vi "average_LockIn.vi"(3 "error in":errorcluster, 4 "Count(mSec)":u32 caption="Sleep between measurements (mSec)", 5 "#AVG":dbl, 6 "Handle In":T2 {"Conn" format="0x%08x"}) -> (0 "Error Out":errorcluster, 1 "output cluster":T1, 2 "Handle Out":T2 {"Conn" format="0x%08x"})   [LabVIEW 2014]
uses:
  <instrlib>/Zurich Instruments LabOne/Public/ziTypeHandle.ctl
  <vilib>/express/express arith-compare/Formula/XNode/ExpressFormulaBlockNode.xnode
  <vilib>/Analysis/NI_AALBase.lvlib
  <instrlib>/Zurich Instruments LabOne/Zurich Instruments LabOne.lvlib
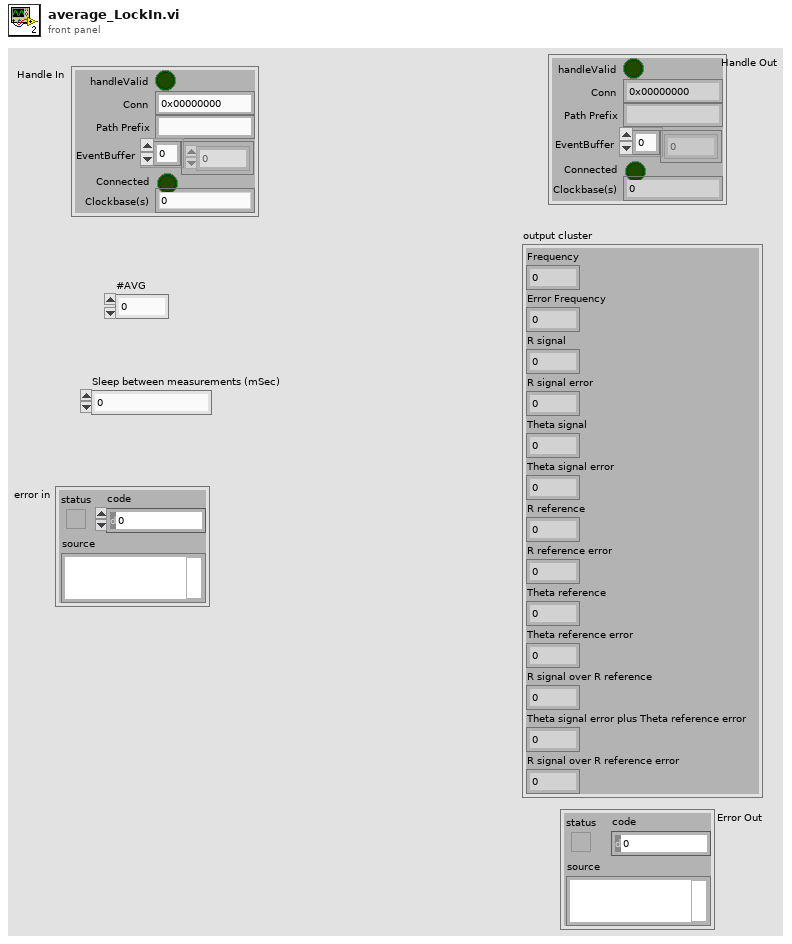
[diagram p1: front panel]
types:
  T1 = cluster{"Frequency":dbl, "Error Frequency ":dbl, "R signal":dbl, "R signal error":dbl, "Theta signal":dbl, "Theta signal error":dbl, "R reference":dbl, "R reference error":dbl, "Theta reference":dbl, "Theta reference error":dbl, "R signal over R reference":dbl, "Theta signal error plus Theta reference error":dbl, "R signal over R reference error":dbl}
  T2 = typedef "Zurich Instruments LabOne.lvlib/ziTypeHandle.ctl" = cluster{"handleValid":bool, "Conn":u64, "Path Prefix":string, "EventBuffer":u8[], "Connected":bool, "Clockbase(s)":dbl}
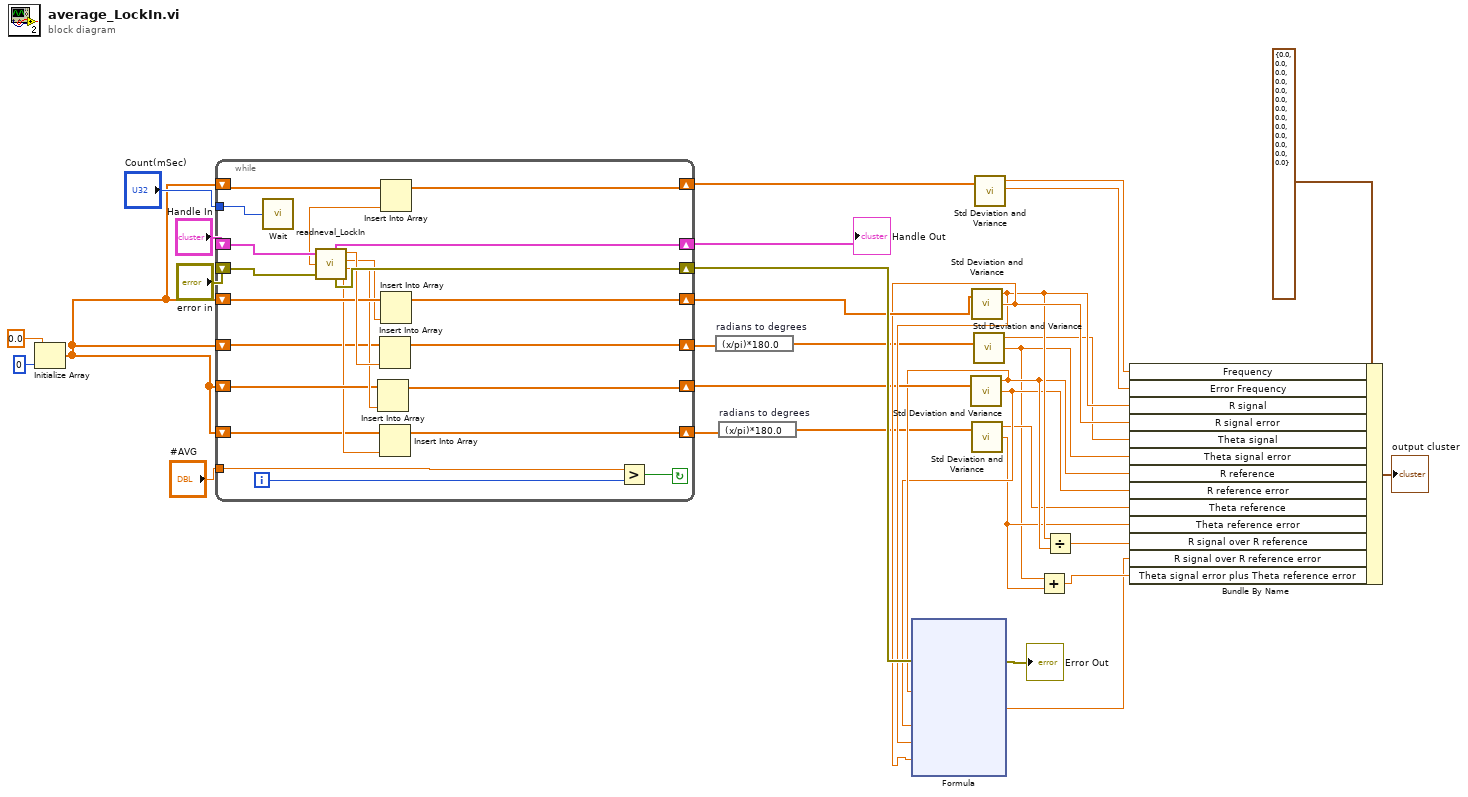
[diagram p0: block diagram]
diagram:
  n1 = Initialize Array(0.0 ("element"), 0 ("dimension size")) -> (w8:dbl[])
  n2 = while {
    shift-right: [w49] -> w24
    shift-left: "error in" -> [w55]
    shift-right: [w53] -> w30
    shift-left: "Handle In" -> [w54]
    tunnel: "#AVG" -> [w51]
    shift-right: [w33] -> w14
    shift-left: w8 -> [w47]
    shift-right: [w45] -> w4
    shift-left: w8 -> [w34]
    shift-right: [w43] -> w20
    shift-left: w8 -> [w44]
    shift-right: [w39] -> w17
    shift-left: w8 -> [w40]
    shift-right: [w36] -> w6
    shift-left: w8 -> [w37]
    tunnel: "Count(mSec)" -> [w35]
    i -> [w50]
    stop <- w52 continue-if-true
    n3 = call "Wait"("Count(mSec)"=w35) -> ()  [unwired: 1 out]
    n4 = call "readneval_LockIn.vi"("error in"=w55, "Handle In"=w54) -> ("Theta reference"=w38:dbl, "Error Out"=w49:errorcluster, "R reference"=w41:dbl, "R signal"=w42:dbl, "Handle Out"=w53:T2, "Theta signal"=w46:dbl, "Freq (Hz)"=w48:dbl)
    n5 = Insert Into Array(array=w40, new element=w41) -> (w39:dbl[])  [unwired: 1 in]
    n6 = Insert Into Array(array=w34, new element=w46) -> (w45:dbl[])  [unwired: 1 in]
    n7 = Insert Into Array(array=w37, new element=w38) -> (w36:dbl[])  [unwired: 1 in]
    n8 = Insert Into Array(array=w47, new element=w48) -> (w33:dbl[])  [unwired: 1 in]
    n9 = Insert Into Array(array=w44, new element=w42) -> (w43:dbl[])  [unwired: 1 in]
    n10 = Greater?(x=w51, y=w50) -> (0:w52:bool)
  }
  "Handle Out" <- w30
  n11 = expression code="(x/pi)*180.0" "radians to degrees"(w4) -> (w3:dbl[])
  n12 = expression code="(x/pi)*180.0" "radians to degrees"(w6) -> (w5:dbl[])
  n13 = call <vilib>:"Std Deviation and Variance.vi"("X"=w17) -> ("mean"=w16:dbl, "standard deviation"=w15:dbl)  [unwired: 1 in, 1 out]
  n14 = call <vilib>:"Std Deviation and Variance.vi"("X"=w20) -> ("mean"=w18:dbl, "standard deviation"=w19:dbl)  [unwired: 1 in, 1 out]
  n15 = xnode "Formula"("R1"=w16, "R1e"=w15, "R2"=w18, "R2e"=w19, "error in (no error)"=w24) -> ("Result"=w25:dbl, "error out"=→"Error Out":errorcluster)
  n16 = call <vilib>:"Std Deviation and Variance.vi"("X"=w5) -> ("mean"=w11:dbl, "standard deviation"=w10:dbl)  [unwired: 1 in, 1 out]
  n17 = call <vilib>:"Std Deviation and Variance.vi"("X"=w3) -> ("mean"=w2:dbl, "standard deviation"=w1:dbl)  [unwired: 1 in, 1 out]
  n18 = call <vilib>:"Std Deviation and Variance.vi"("X"=w14) -> ("mean"=w13:dbl, "standard deviation"=w12:dbl)  [unwired: 1 in, 1 out]
  n19 = Add(x=w1, y=w10) -> (x+y=w26:dbl)
  n20 = Divide(x=w18, y=w16) -> (x/y=w27:dbl)
  n21 = Bundle By Name(cluster=T1 {"Frequency"=0.0, "Error Frequency "=0.0, "R signal"=0.0, "R signal error"=0.0, "Theta signal"=0.0, "Theta signal error"=0.0, "R reference"=0.0, "R reference error"=0.0, "Theta reference"=0.0, "Theta reference error"=0.0, "R signal over R reference"=0.0, "Theta signal error plus Theta reference error"=0.0, "R signal over R reference error"=0.0}, "Frequency"=w13, "Error Frequency"=w12, "R signal"=w18, "R signal error"=w19, "Theta signal"=w2, "Theta signal error"=w1, "R reference"=w16, "R reference error"=w15, "Theta reference"=w11, "Theta reference error"=w10, "R signal over R reference"=w27, "R signal over R reference error"=w25, "Theta signal error plus Theta reference error"=w26) -> (→"output cluster":T1)
